vi "33250A_Kharon.vi"(9 "Output Load Configuration":T1={"Output Load Impedence"=enum."50 Ohms", "Load value (ohms)"=50.0} {"Load value (ohms)" min=1.0 max=10000.0 step=1.0 format="%.0p"}, 10 "Standard Waveform Configuration":T3={"Frequency (Hz)"=1000.0, "Waveform Function"=1, "DC Offset (V)"=0.0, "Unit"=0, "Amplitude (V)"=1.0, "Duty cycle (%)"=50.0} {"Duty cycle (%)" min=0.002 max=99.999 step=0.001 format="%.3p"; "Amplitude (V)" min=0.001 max=20.0 format="%#_6p"; "Unit" items=["Vpp", "Vrms", "dB"]; "DC Offset (V)" min=-10.0 max=10.0 format="%#_6p"; "Waveform Function" items=["DC", "Sine", "Square", "Triangle", "Ramp", "Pulse", "Noise", "Sinc", "Negative Ramp", "Exponential Rise", "Exponential Fall", "Cardiac"]; "Frequency (Hz)" min=1e-06 max=80000000.0 format="%#_6p"}, 11 "Instrument Address":refnum<visa-resource-name>) -> (0 "error out":errorcluster, 8 "error in":errorcluster)   [LabVIEW 2019]
uses:
  <userlib>/_TI-LA/Instr Drivers/Signal Generator/33XXX/Driver/EasyIO/Typedef/33XXX Standard Waveform Configuration.ctl
  <userlib>/_TI-LA/Instr Drivers/Signal Generator/33XXX/Driver/EasyIO/Typedef/33XXX Waveform Function.ctl
  <userlib>/_TI-LA/Instr Drivers/Signal Generator/33XXX/Driver/EasyIO/Typedef/33XXX Waveform Unit.ctl
  <userlib>/_TI-LA/Instr Drivers/Signal Generator/33XXX/Modules/33XXX Modules.lvlib
  <userlib>/_TI-LA/Instr Drivers/Signal Generator/33XXX/Driver/33XXX.lvlib
  <userlib>/_TI-LA/Instr Drivers/Signal Generator/33XXX/Driver/EasyIO/Typedef/33XXX Output Load Termination.ctl
  <userlib>/_TI-LA/Instr Drivers/Signal Generator/33XXX/Driver/EasyIO/Typedef/33XXX Output Load.ctl
panel:
  in  "Enable Output?":bool=TRUE
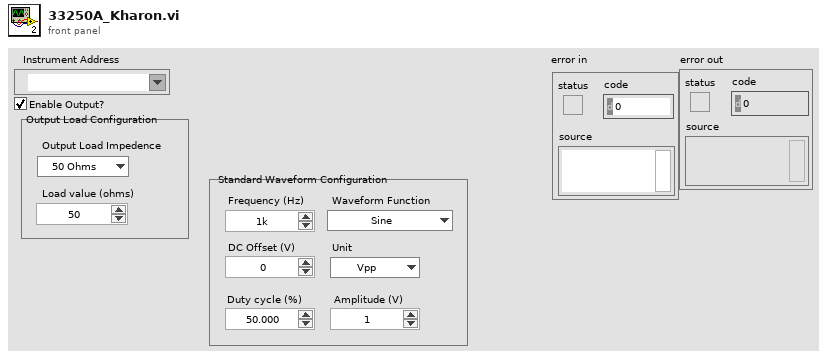
[diagram p1: front panel]
types:
  T1 = typedef "33XXX.lvlib/33XXX Output Load.ctl" = cluster{"Output Load Impedence":T2, "Load value (ohms)":dbl}
  T2 = typedef "33XXX.lvlib/33XXX Output Load Termination.ctl" = enum16{"50 Ohms", "High Z", "User Defined"}
  T3 = typedef "33XXX.lvlib/33XXX Standard Waveform Configuration.ctl" = cluster{"Frequency (Hz)":dbl, "Waveform Function":T4, "DC Offset (V)":dbl, "Unit":T5, "Amplitude (V)":dbl, "Duty cycle (%)":dbl}
  T4 = typedef "33XXX.lvlib/33XXX Waveform Function.ctl" = u16
  T5 = typedef "33XXX.lvlib/33XXX Waveform Unit.ctl" = u16
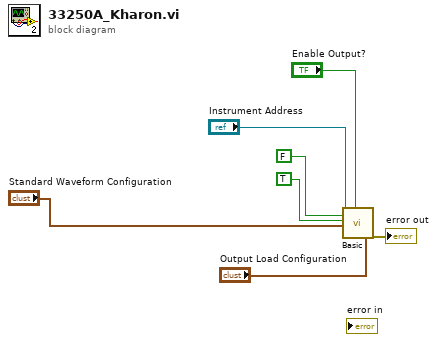
[diagram p0: block diagram]
diagram:
  n1 = call <userlib>:"Basic.vi"("Instrument Address"="Instrument Address", "Reset?"=FALSE, "ID Query?"=TRUE, "Standard Waveform Configuration"="Standard Waveform Configuration", "Enable Output?"="Enable Output?", "Output Load Configuration"="Output Load Configuration") -> ("error out"=→"error out":errorcluster)  [unwired: 11 in, 2 out]
